vi "File.Rotate.Manager - Core.vi"(9 "Q Name":string="FileRotate", 11 "Config Folder":path) -> ()   [LabVIEW 2024, in "KATE_Lib.lvlib" / "File Utils.lvlib" / "File.Rotate.lvclass"]
uses:
  File.Rotate.lvclass
  File.Rotate.Rotation Task Item.ctl
  Queues/Queue Utils.lvlib
  Scheduler/Scheduler.lvlib
  File Utils.lvlib
panel:
  in  "Tab Control":enum32{"Inputs", "Front Panel"}(tab)=enum."Front Panel"
  out "Busy":bool
  out "Rotation Config":T1[](array[typedef]) {"LastRotate" format="%<%X\n%x>T"}
  # "File Rotation"
  # "Name/Interval                                                                                             Folder and Max Counts"
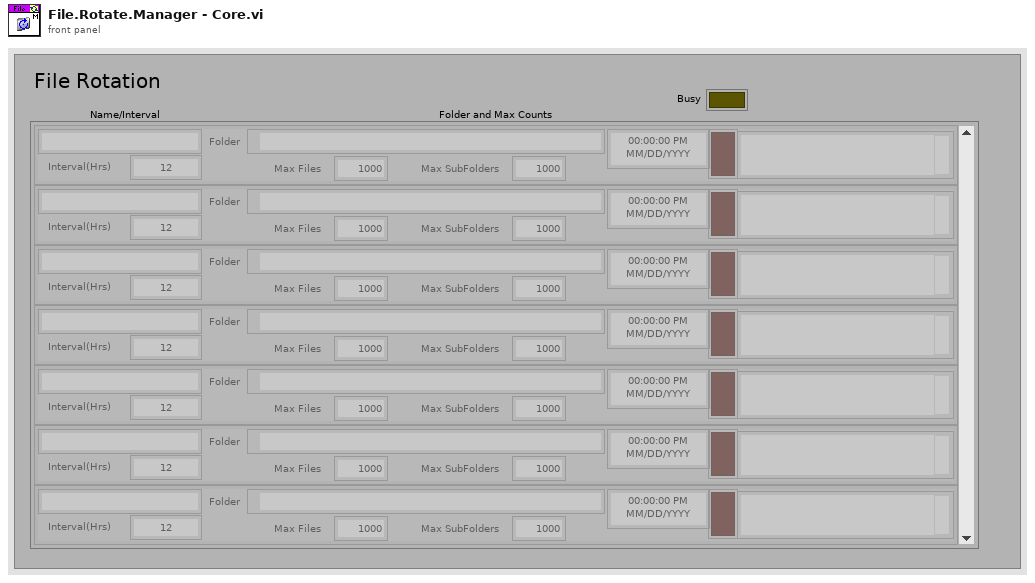
[diagram p1: front panel]
types:
  T1 = typedef "KATE_Lib.lvlib/File Utils.lvlib/File.Rotate.lvclass/File.Rotate.Rotation Task Item.ctl" = cluster{"Name":string, "Interval":dbl, "Folder":path, "Max Files":i32, "Max SubFolders":i32, "LastRotate":timestamp, "Error":bool, "Status":string}
  T2 = cluster{"Config Folder":path, "Rotate":refnum<class "File.Rotate.lvclass">}
  T3 = cluster{"Name":string, "Interval":dbl, "Folder":path, "Max Files":i32, "Max SubFolders":i32, "LastRotate":timestamp, "Error":bool, "Status":string}[]
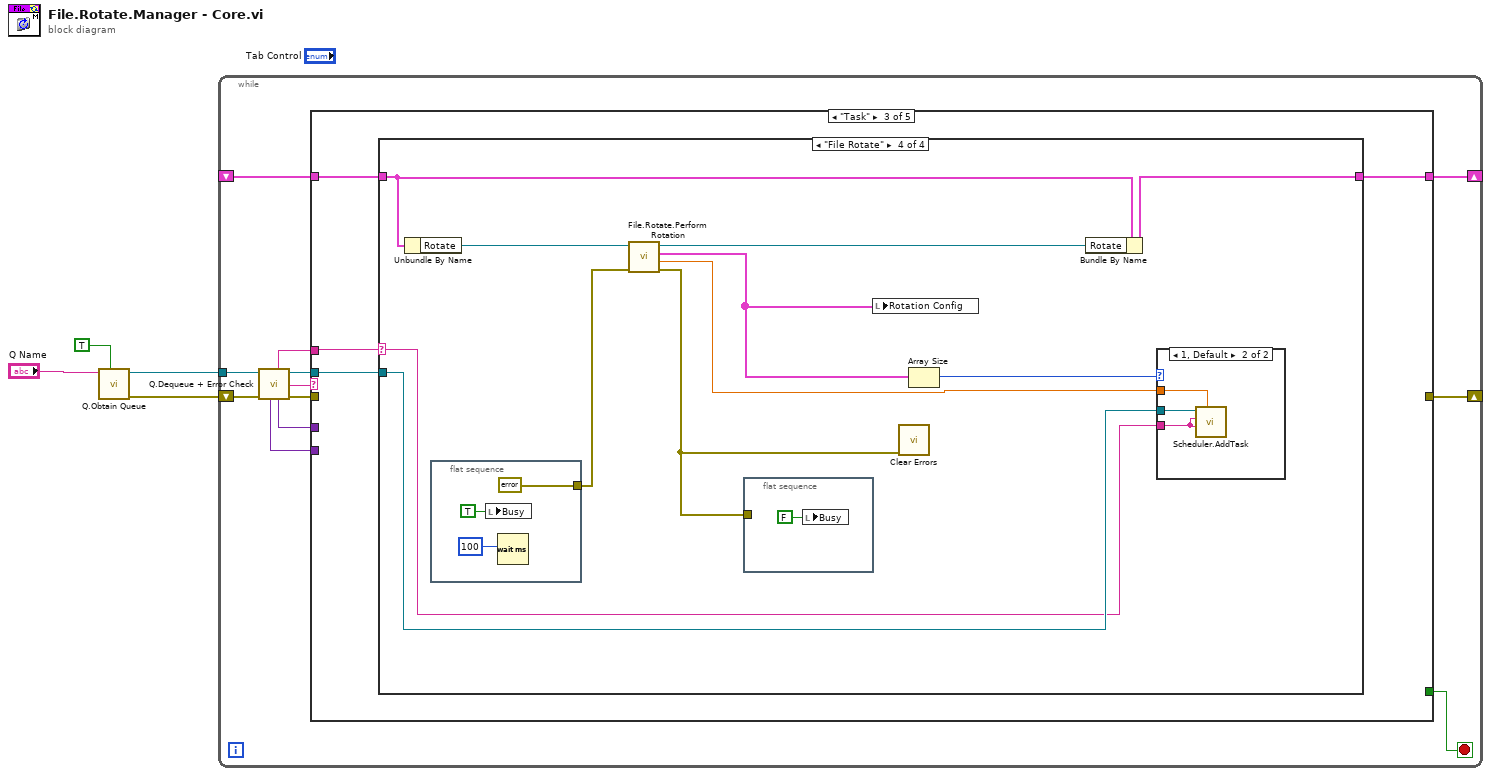
[diagram p0: block diagram]
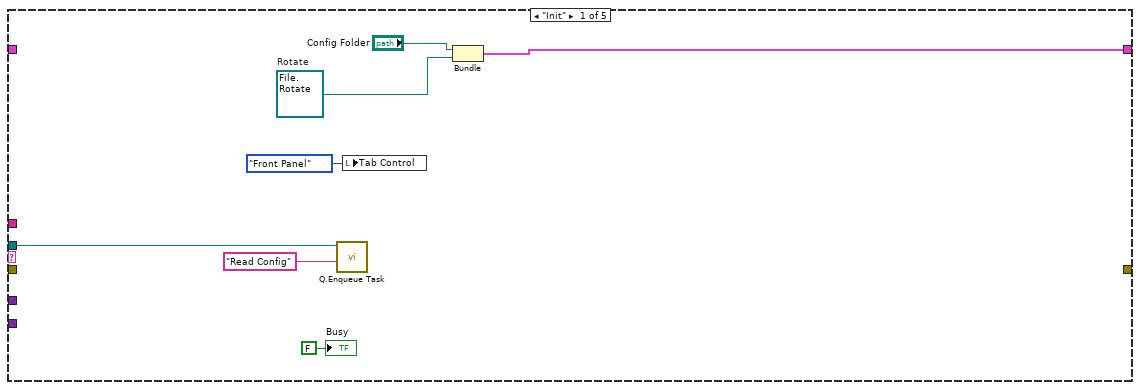
[diagram p2: hidden frame]
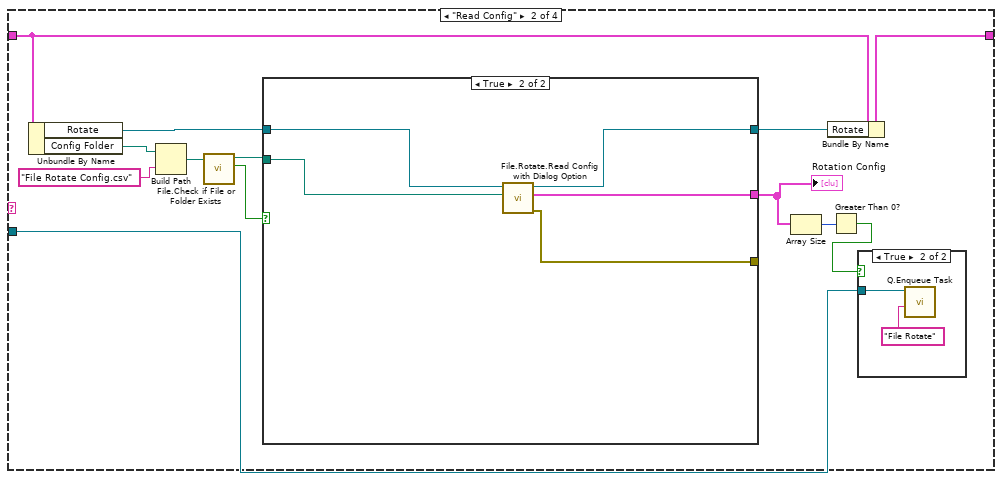
[diagram p5: hidden frame]
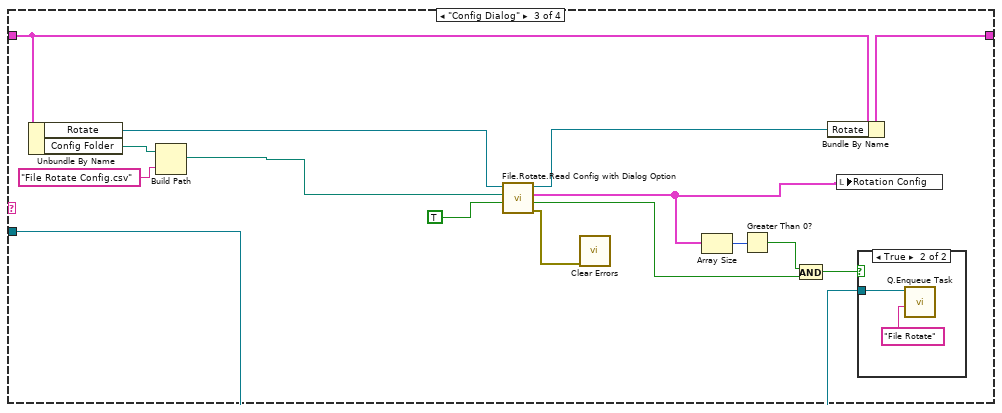
[diagram p8: hidden frame]
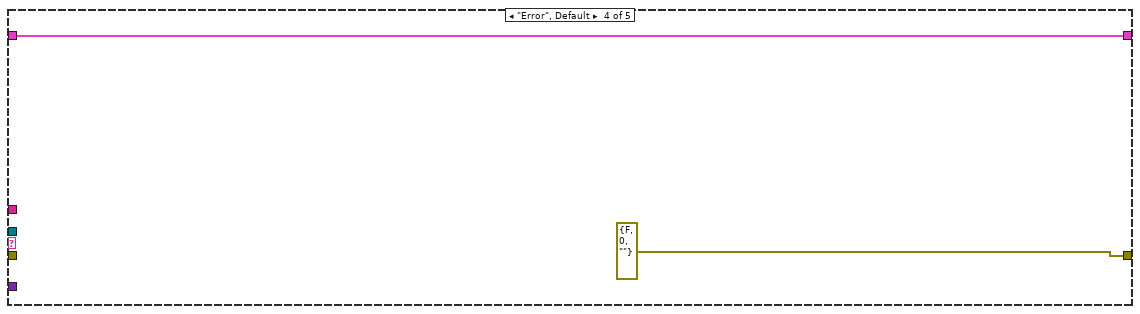
[diagram p11: hidden frame]
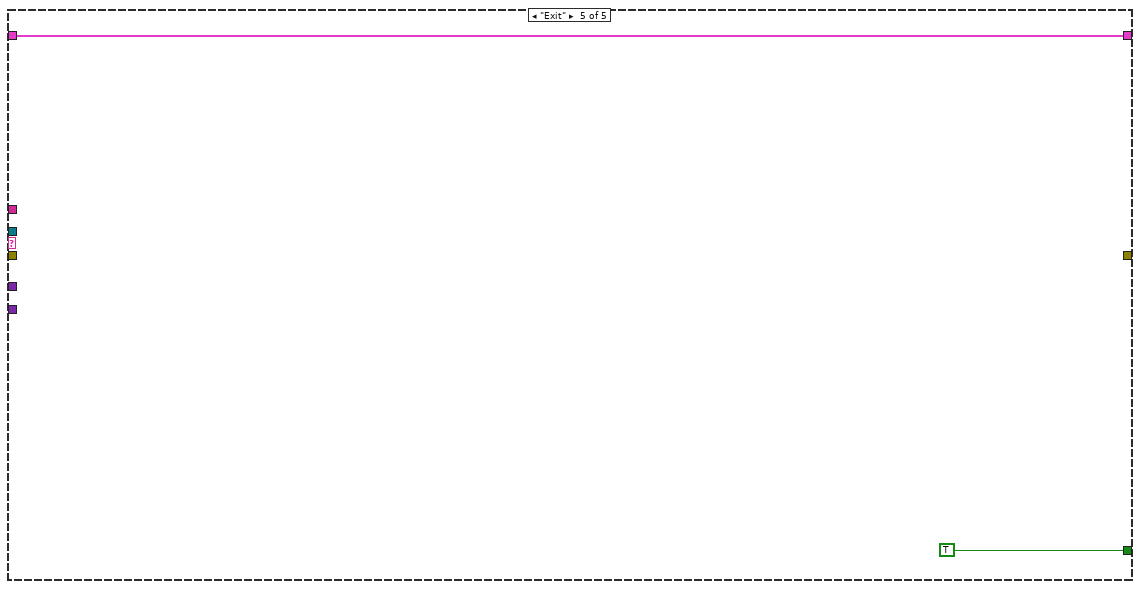
[diagram p12: hidden frame]
diagram:
  n1 = call "Q.Obtain Queue.vi"("Enqueue Init"=TRUE, "Q Name"="Q Name") -> ("error out"=w4:errorcluster, "Q Out"=w1:refnum<queue>)  [unwired: 7 in, 1 out]
  n2 = while {
    shift-right: [w7] -> _
    shift-left: w4 -> [w16]
    tunnel: w1 -> [w9]
    shift-right: [w5] -> _
    shift-left: _ -> [w6]
    stop <- w8 stop-if-true
    n3 = call "Q.Dequeue + Error Check.vi"("Error In"=w16, "Q In"=w9) -> ("error out"=w15:errorcluster, "Cmd"=w14:string, "Q Out"=w13:refnum<queue>, "Data1"=w11:variant, "Sub"=w12:string, "Data2"=w10:variant)  [unwired: 4 in]
    n4 = case shown="\"Task\"" w14 {
      tunnel: w15 -> [_ _ _ _ _]
      tunnel: w13 -> [w21 _ w25 _ _]
      tunnel: w12 -> [_ _ w28 _ _]
      tunnel: w11 -> [_ _ _ _ _]
      tunnel: w10 -> [_ _ _ _ _]
      tunnel: [_ _ _ _ TRUE] -> w8
      tunnel: [_ _ _ errorcluster {"status"=FALSE, "code"=0, "source"=""} ("error constant") _] -> w7
      tunnel: w6 -> [_ w24 w27 w86 w88]
      tunnel: [w22 w24 w26 w86 w88] -> w5
      frame "Init" {
        w19 = refnum<class "File.Rotate.lvclass"> refnum  # Rotate
        n5 = call "Q.Enqueue Task.vi"("Task Name"="Read Config", "Q In"=w21) -> ()  [unwired: 8 in, 2 out]
        n6 = local write "Tab Control"(enum32{"Inputs", "Front Panel"}."Front Panel" ("Tab Control")) -> ()
        n7 = Bundle("Config Folder"="Config Folder", "Rotate"=w19) -> (w22:T2)  [unwired: 1 in]
        "Busy" <- FALSE ("Busy")
      }
      frame "Reset" {
      }
      frame "Task" {
        n8 = case shown="\"File Rotate\"" w28 {
          selector: w28 -> [_ _ _ w75]
          tunnel: w27 -> [w29 w39 w62 w77]
          tunnel: [w29 w40 w63 w78] -> w26
          tunnel: w25 -> [_ w36 w59 w76]
          frame Default {
          }
          frame "Read Config" {
            n9 = Unbundle By Name(w39) -> ("Rotate"=w31:refnum<class "File.Rotate.lvclass">, "Config Folder"=w42:path)
            n10 = Build Path(base path=w42, name or relative path="File Rotate Config.csv") -> (appended path=w34:path)
            n11 = call "File.Check if File or Folder Exists.vi"("Path"=w34) -> ("Exists"=w32:bool, "Dup Path"=w33:path)  [unwired: 6 in, 3 out]
            n12 = case shown="True" w32 {
              tunnel: w33 -> [_ w49]
              tunnel: [w45 w48] -> w38
              tunnel: w31 -> [w45 w50]
              tunnel: [_ w47] -> w30
              tunnel: [_ w46] -> _
              frame False {
              }
              frame True {
                n13 = call "File.Rotate.Read Config with Dialog Option.vi"("Config File"=w49, "File.Rotate in"=w50) -> ("error out"=w46:errorcluster, "Tasks"=w47:T1[], "File.Rotate out"=w48:refnum<class "File.Rotate.lvclass">)  [unwired: 6 in, 1 out]
              }
            }
            "Rotation Config" <- w30
            n14 = Array Size(array=w30) -> (size(s)=w37:i32)
            n15 = Bundle By Name(cluster=w39, "Rotate"=w38) -> (w40:T2)
            n16 = Greater Than 0?(x=w37) -> (x > 0?=w35:bool)
            n17 = case shown="True" w35 {
              tunnel: w36 -> [_ w43]
              frame False {
              }
              frame True {
                n18 = call "Q.Enqueue Task.vi"("Task Name"="File Rotate", "Q In"=w43) -> ()  [unwired: 8 in, 2 out]
              }
            }
          }
          frame "Config Dialog" {
            n19 = Unbundle By Name(w62) -> ("Rotate"=w58:refnum<class "File.Rotate.lvclass">, "Config Folder"=w65:path)
            n20 = Build Path(base path=w65, name or relative path="File Rotate Config.csv") -> (appended path=w56:path)
            n21 = call "File.Rotate.Read Config with Dialog Option.vi"("Dialog"=TRUE, "Config File"=w56, "File.Rotate in"=w58) -> ("error out"=w54:errorcluster, "Saved"=w53:bool, "Tasks"=w57:T1[], "File.Rotate out"=w61:refnum<class "File.Rotate.lvclass">)  [unwired: 5 in]
            n22 = call <vilib>:"Clear Errors.vi"("error in (no error)"=w54) -> ()  [unwired: 5 in, 2 out]
            n23 = Array Size(array=w57) -> (size(s)=w60:i32)
            n24 = Greater Than 0?(x=w60) -> (x > 0?=w52:bool)
            n25 = And(x=w52, y=w53) -> (x .and. y?=w51:bool)
            n26 = Bundle By Name(cluster=w62, "Rotate"=w61) -> (w63:T2)
            n27 = local write "Rotation Config"(w57) -> ()
            n28 = case shown="True" w51 {
              tunnel: w59 -> [_ w66]
              frame False {
              }
              frame True {
                n29 = call "Q.Enqueue Task.vi"("Task Name"="File Rotate", "Q In"=w66) -> ()  [unwired: 8 in, 2 out]
              }
            }
          }
          frame "File Rotate" {
            n30 = Unbundle By Name(w77) -> ("Rotate"=w73:refnum<class "File.Rotate.lvclass">)
            n31 = flat-sequence {
              tunnel: [errorcluster {"status"=FALSE, "code"=0, "source"=""} ("error constant")] -> w68
              frame #0 {
                n32 = local write "Busy"(TRUE ("Busy")) -> ()
                n33 = Wait (ms)(milliseconds to wait=u32 100 ("millisecond timer value")) -> ()  [unwired: 1 out]
              }
            }
            n34 = call "File.Rotate.Perform Rotation.vi"("error in (no error)"=w68, "File.Rotate in"=w73) -> ("error out"=w69:errorcluster, "Next Check(s)"=w70:dbl, "Task Status"=w71:T3, "File.Rotate out"=w72:refnum<class "File.Rotate.lvclass">)  [unwired: 6 in]
            n35 = flat-sequence {
              tunnel: w69 -> [_]
              frame #0 {
                n36 = local write "Busy"(FALSE ("Busy")) -> ()
              }
            }
            n37 = local write "Rotation Config"(w71) -> ()
            n38 = call <vilib>:"Clear Errors.vi"("error in (no error)"=w69) -> ()  [unwired: 5 in, 2 out]
            n39 = Array Size(array=w71) -> (size(s)=w74:i32)
            n40 = Bundle By Name(cluster=w77, "Rotate"=w72) -> (w78:T2)
            n41 = case shown="1, Default" w74 {
              tunnel: w76 -> [_ w85]
              tunnel: w70 -> [_ w84]
              tunnel: w75 -> [_ w83]
              frame 0 {
              }
              frame 1, Default {
                n42 = call "Scheduler.AddTask.vi"("Interval(s)"=w84, "Task Name"=w83, "Sched Name"=w83, "Q In"=w85) -> ()  [unwired: 6 in, 2 out]
              }
            }
          }
        }
      }
      frame "Error", Default {
      }
      frame "Exit" {
      }
    }
  }
